vi "MTM2_getNextSample_forceBalance.vi"(8 "error in (no error)":errorcluster, 11 "forceBalance_Ctl":T1) -> (0 "error out":errorcluster, 2 "function return":i32, 3 "forceBalance_Ctl out":T1)   [LabVIEW 2018, in "SALLV_MTM2.lvlib"]
doc: "int MTM2_shm_getNextSample_forceBalanceLV(MTM2_forceBalanceLV *forceBalance_Ctl );"
uses:
  DataTypes/forceBalance.ctl
  SALLV_MTM2.lvlib
  SALLV_MTM2.so
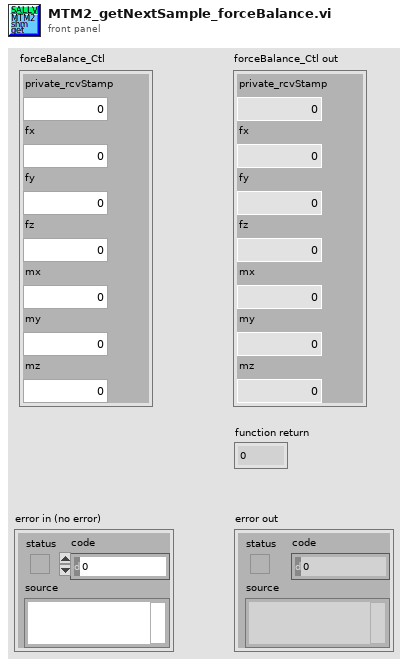
[diagram p1: front panel]
types:
  T1 = typedef "SALLV_MTM2.lvlib/forceBalance.ctl" = cluster{"private_rcvStamp":dbl, "fx":dbl, "fy":dbl, "fz":dbl, "mx":dbl, "my":dbl, "mz":dbl}
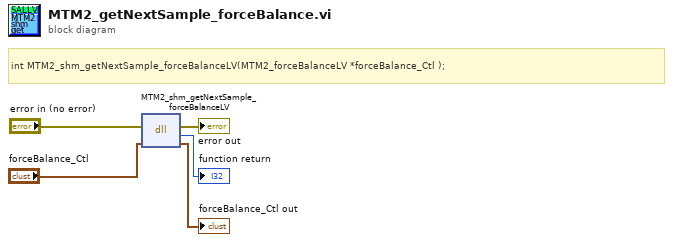
[diagram p0: block diagram]
diagram:
  # "int MTM2_shm_getNextSample_forceBalanceLV(MTM2_forceBalanceLV *forceBalance_Ctl );"
  n1 = dll-call lib="home/ttsai/Documents/salTestLabViewApi/SALLV_MTM2/SALLV_MTM2.*" fn="MTM2_shm_getNextSample_forceBalanceLV"(error in="error in (no error)", "forceBalance_Ctl"="forceBalance_Ctl") -> (error out=→"error out":errorcluster, →"function return":i32, "forceBalance_Ctl"=→"forceBalance_Ctl out":T1)  [unwired: 2 in, 1 out]
